vi "getAttributesPublic.vi"(0 "reference in":refnum<class "VINode.lvclass">, 5 "error in (no error)":errorcluster) -> (14 "reference out":refnum<class "VINode.lvclass">, 15 "methods":refnum<class "MultiLineString.lvclass">, 19 "error out":errorcluster)   [LabVIEW 2014]
doc: "public MultiLineString getAttributes()"
uses:
  <resource>/Framework/Providers/Open_GDS/UML/VINode_class/VINode.lvclass
  <resource>/Framework/Providers/Open_GDS/UML/MultiLineString_class/MultiLineString.lvclass
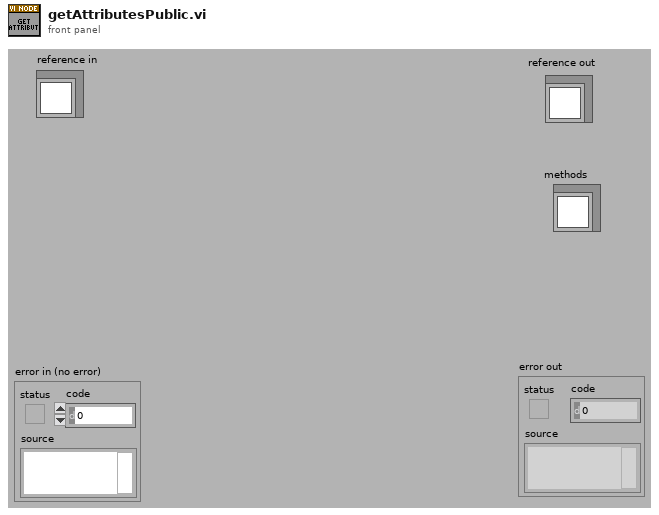
[diagram p1: front panel]
types:
  T1 = typedef "VINode.lvclass/ObjectAttributes.ctl" = cluster{"midHeight":dbl, "botHeight":dbl, "Name":refnum<class "MultiLineString.lvclass">, "DEFAULT_COMPARTMENT_HEIGHT":i32, "DEFAULT_WIDTH":i32, "DEFAULT_HEIGHT":i32, "ClassPath":path, "Icon":u8[][]}
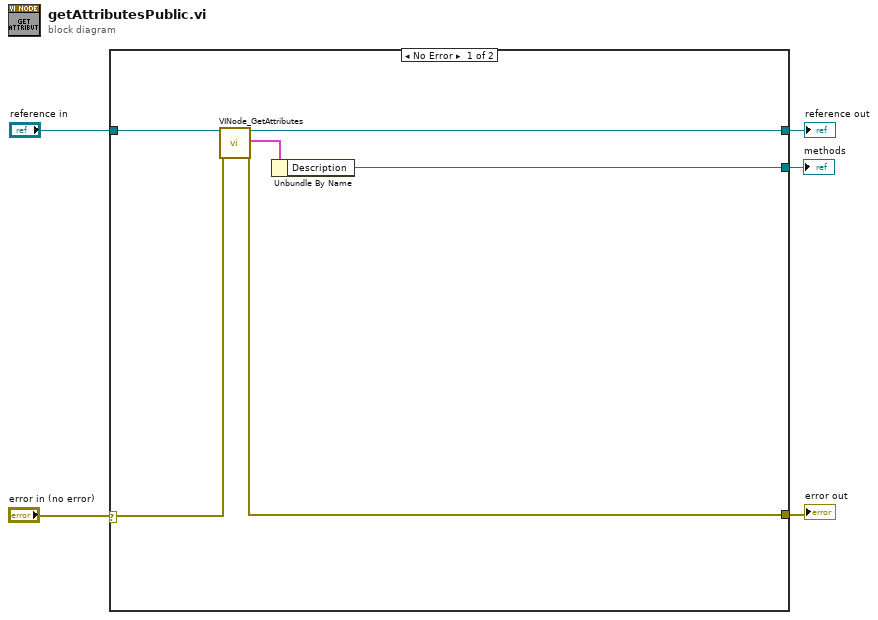
[diagram p0: block diagram]
diagram:
  n1 = case shown="No Error" "error in (no error)" {
    selector: "error in (no error)" -> [w7 w12]
    tunnel: "reference in" -> [w11 w13]
    tunnel: [w10 w12] -> w4
    tunnel: [w9 w13] -> w3
    tunnel: [w8 _] -> w1
    frame No Error {
      n2 = call <resource>:"VINode_GetAttributes.vi"("reference in"=w11, "error in (no error)"=w7) -> ("reference out"=w9:refnum<class "VINode.lvclass">, "Data"=w6:T1, "error out"=w10:errorcluster)  [unwired: 1 in, 14 out]
      n3 = Unbundle By Name(w6) -> ("Description"=w8:refnum<class "MultiLineString.lvclass">)
    }
    frame Error {
    }
  }
  "reference out" <- w3
  "error out" <- w4
  "methods" <- w1
